vi "Main.vi"() -> ()   [LabVIEW 2016]
uses:
  SubVIS/MainSteps.ctl
  <vilib>/Utility/config.llb/Write Key (String).vi
  <vilib>/Utility/config.llb/Write Key (Double).vi
  <vilib>/Utility/config.llb/NI_LVConfig.lvlib
panel:
  out "全局图片":bool=TRUE
  out "新值":enum32{"三角形", "圆形", "正方形"}(ring)
  out "Status":bool
  in  "状态":string
  in  "标定":bool
  in  "停止":bool
  in  "运行":bool
  out "Image":T1(plugin-control)
  in  "选项卡控件":enum32{"三角形", "圆形", "正方形"}(tab)
  in  "Trangle保存":bool
  in  "Trangle打开":bool
  in  "Trangle参考":bool
  in  "多列列表框":i32(listbox)
  in  "Trangle处理":bool
  in  "Point1":cluster{"伺服X":dbl, "伺服Y":dbl}
  in  "Point2":cluster{"伺服X":dbl, "伺服Y":dbl}
  in  "Point3":cluster{"伺服X":dbl, "伺服Y":dbl}
  in  "Mark":cluster{"伺服X":dbl, "伺服Y":dbl}
  in  "半径R":dbl
  in  "Circle参考":bool
  in  "Circle打开":bool
  in  "多列列表框":i32(listbox) caption="圆形"
  in  "Circle保存":bool
  in  "Circle处理":bool
  in  "Mark":cluster{"伺服X":dbl, "伺服Y":dbl}
  in  "Mark":cluster{"伺服X":dbl, "伺服Y":dbl}
  in  "Point4":cluster{"伺服X":dbl, "伺服Y":dbl}
  in  "Point3":cluster{"伺服X":dbl, "伺服Y":dbl}
  in  "Point2":cluster{"伺服X":dbl, "伺服Y":dbl}
  in  "Point1":cluster{"伺服X":dbl, "伺服Y":dbl}
  in  "Square处理":bool
  in  "多列列表框":i32(listbox) caption="正方形"
  in  "Square参考":bool
  in  "Square打开":bool
  in  "Square保存":bool
  # "湖南工业大学毕设视觉平台"
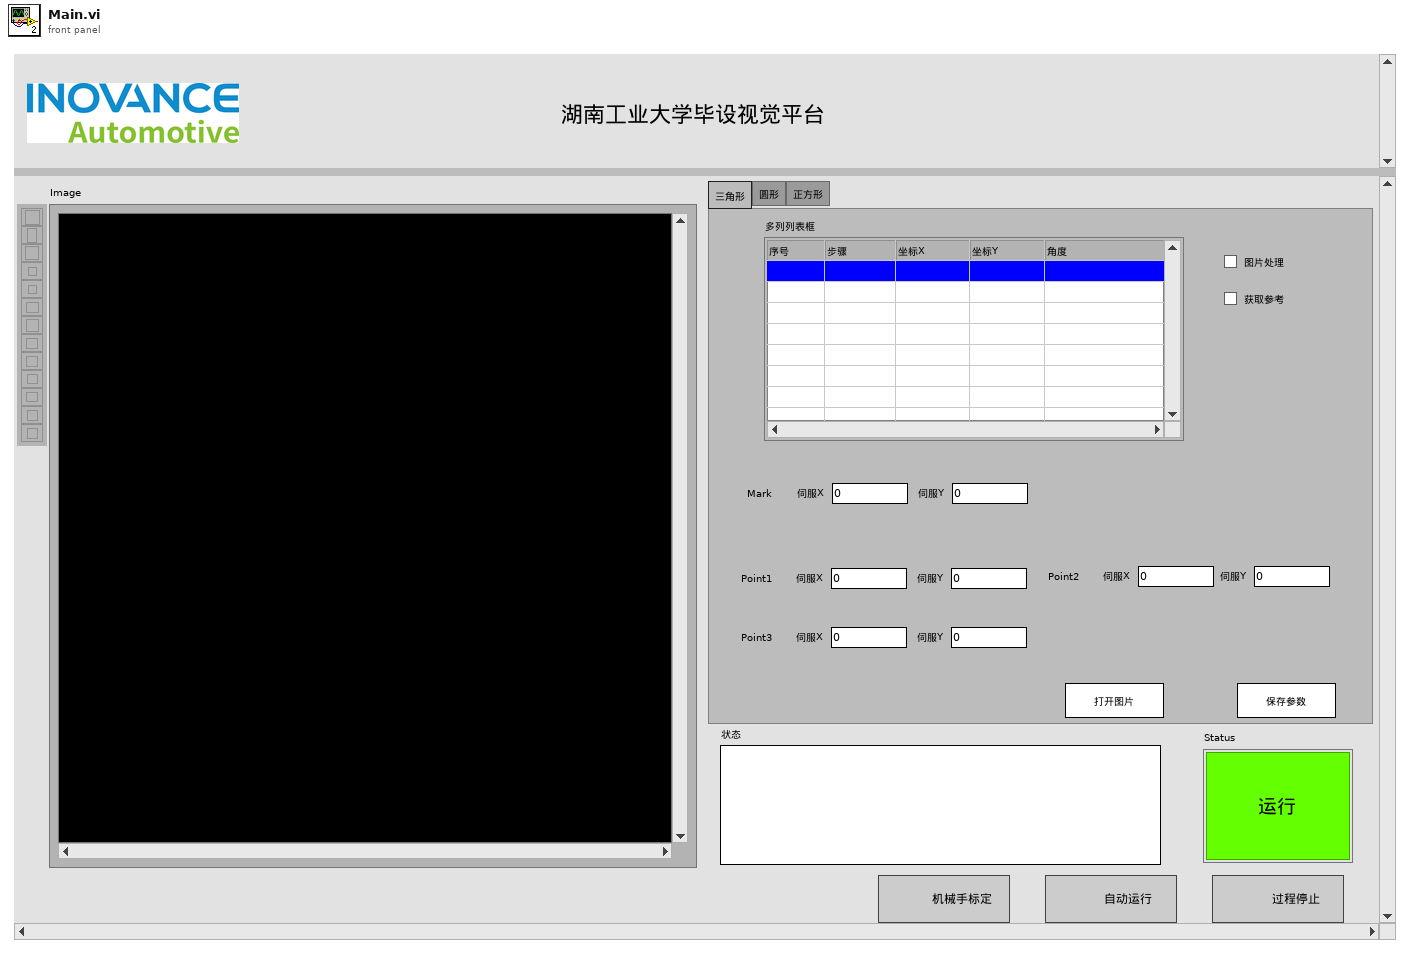
[diagram p1: front panel]
types:
  T1 = typedef "IMAQ Image.ctl" = refnum<image>
  T2 = typedef "MainSteps.ctl" = enum16{"Nothing", "Initial", "ReadConfig", "OpenPicture", "PicturePro", "SaveRefer", "SaveParam", "AutoRun", "Exit"}
  T3 = typedef "Image Type" = u32
  T4 = typedef "NI_LVConfig.lvlib/Config Data RefNum.ctl" = refnum<k1>
  T5 = cluster{"Center (Pixels)":cluster{"X":sgl, "Y":sgl}, "Radius (Pixels)":dbl, "Center (Real-World)":cluster{"X":sgl, "Y":sgl}, "Radius (Real-World)":dbl, "Roundness (Real-World)":dbl, "Average Strength":dbl, "Average SNR (dB)":dbl}
  T6 = cluster{"Position":cluster{"x":sgl, "y":sgl}, "Angle":sgl, "Scale":sgl, "Score":sgl, "Bounding Box":cluster{"x":sgl, "y":sgl}[]}[]
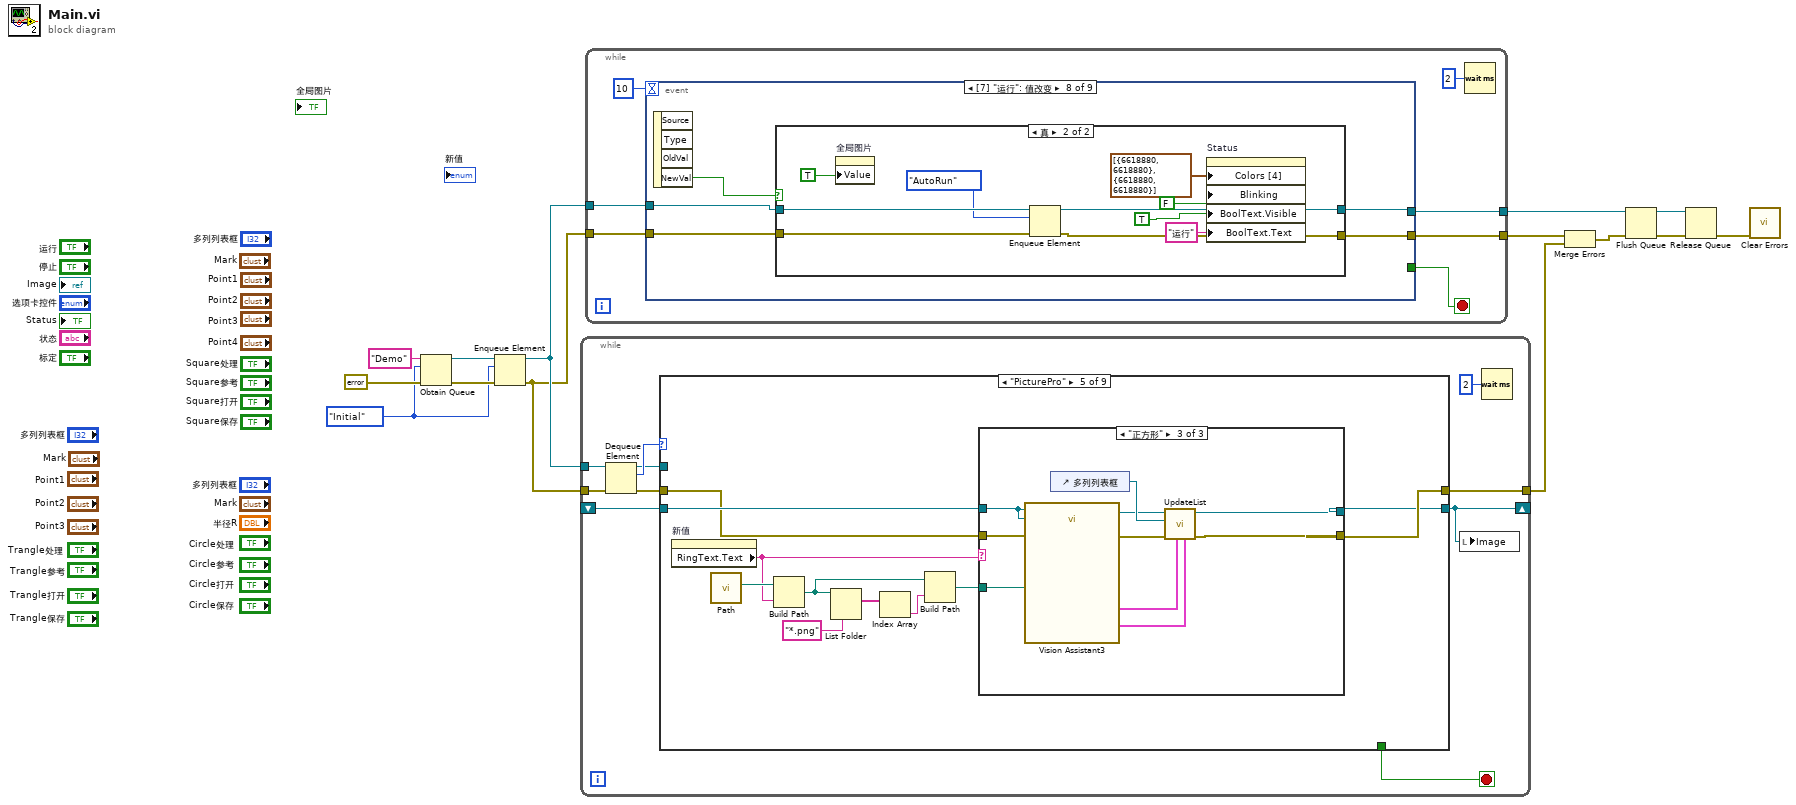
[diagram p0: block diagram]
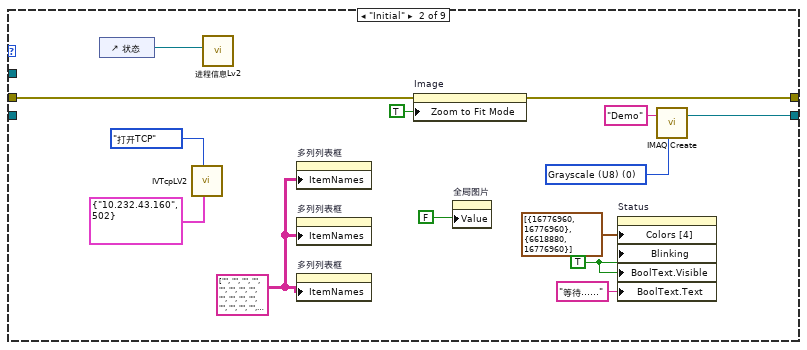
[diagram p3: hidden frame]
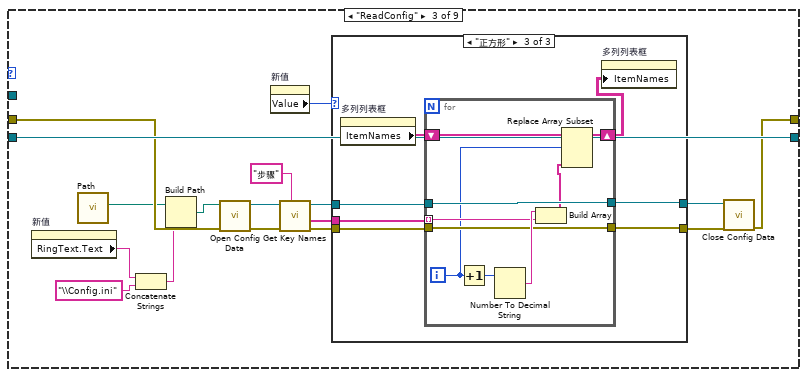
[diagram p4: hidden frame]
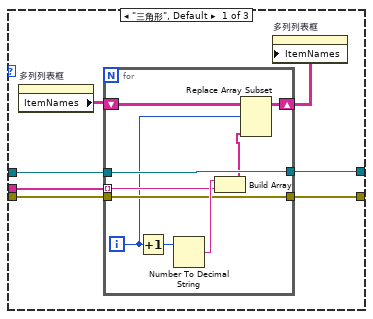
[diagram p5: hidden frame]
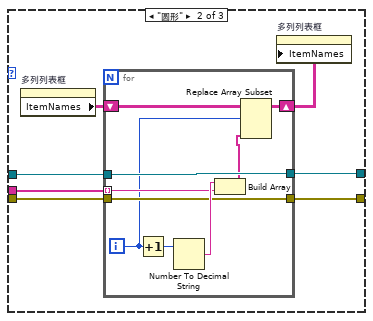
[diagram p6: hidden frame]
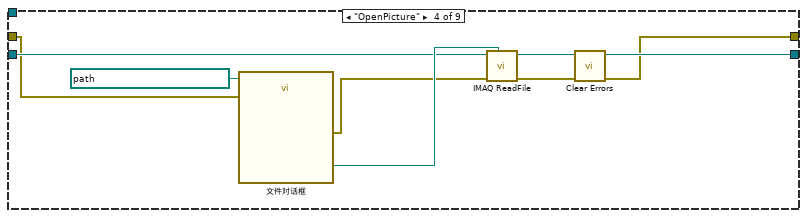
[diagram p7: hidden frame]
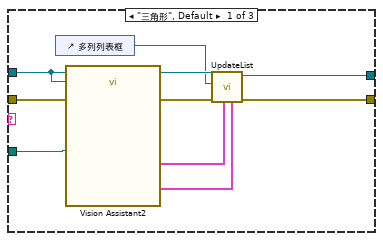
[diagram p8: hidden frame]
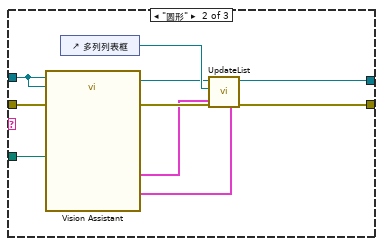
[diagram p9: hidden frame]
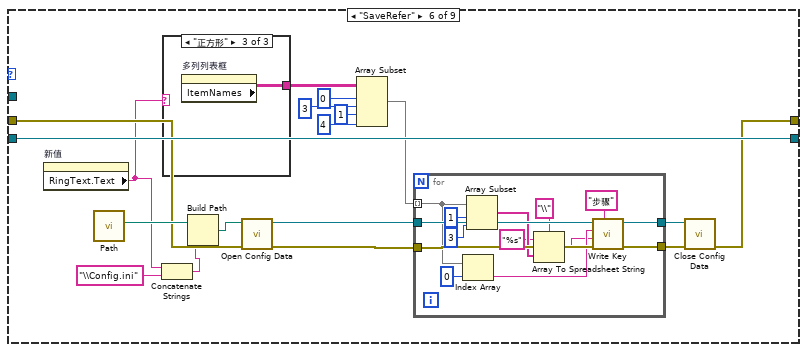
[diagram p10: hidden frame]
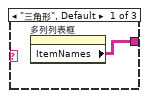
[diagram p11: hidden frame]
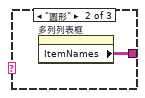
[diagram p12: hidden frame]
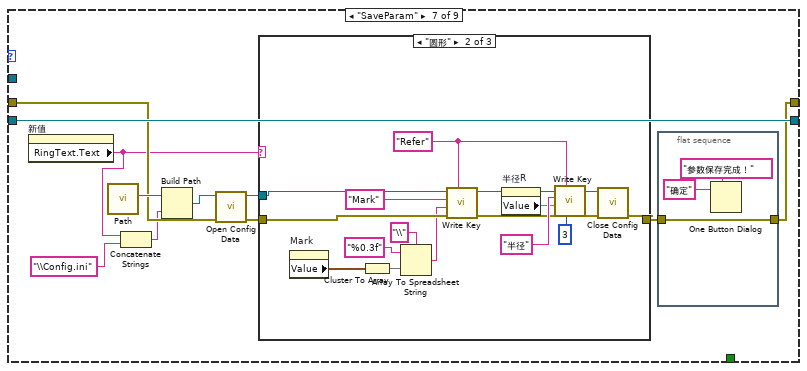
[diagram p13: hidden frame]
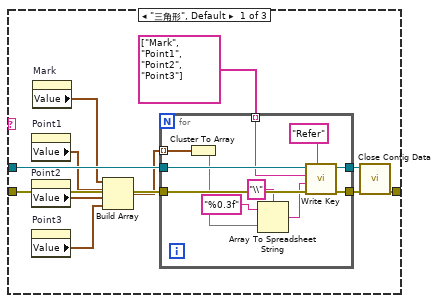
[diagram p14: hidden frame]
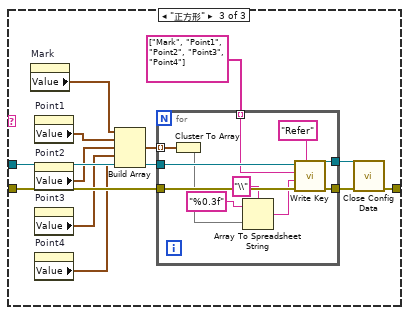
[diagram p15: hidden frame]
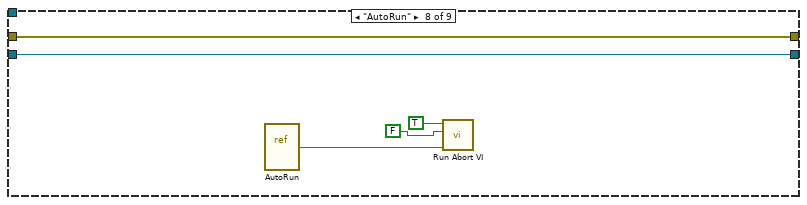
[diagram p16: hidden frame]
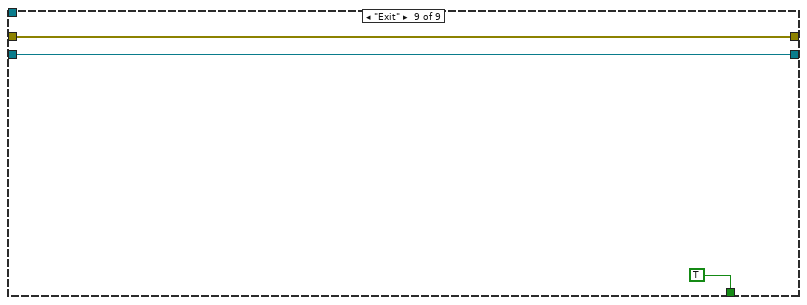
[diagram p17: hidden frame]
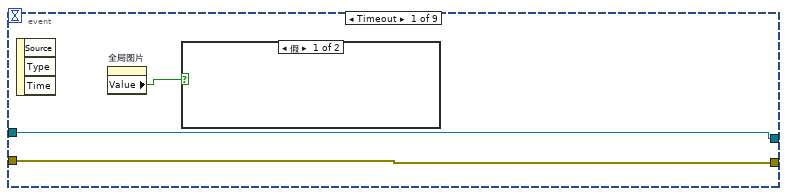
[diagram p18: hidden frame]
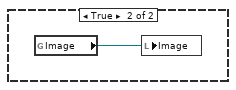
[diagram p19: hidden frame]
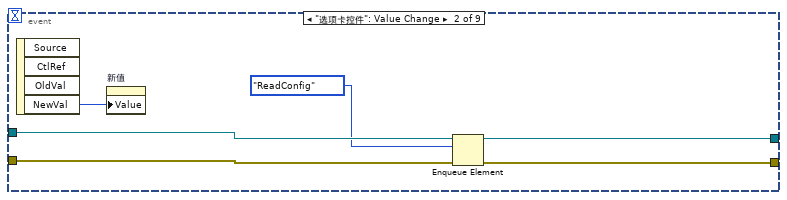
[diagram p20: hidden frame]
diagram:
  w9 = MainSteps."Initial"
  n1 = Obtain Queue(name (unnamed)="Demo" ("名称（未命名）"), element data type=w9, error in (no error)=errorcluster {"status"=FALSE, "code"=0, "source"=""} ("错误输入（无错误）")) -> (queue out=w13:refnum<queue>, error out=w12:errorcluster)  [unwired: 2 in, 1 out]
  n2 = Enqueue Element(queue=w13, element=w9, error in (no error)=w12) -> (queue out=w10:refnum<queue>, error out=w8:errorcluster)  [unwired: 1 in, 1 out]
  n3 = while {
    tunnel: w8 -> [w24]
    tunnel: w10 -> [w23]
    shift-right: [w16] -> _
    shift-left: _ -> [w19]
    tunnel: [w18] -> w6
    stop <- w17 stop-if-true
    n4 = Dequeue Element(queue=w23, error in (no error)=w24) -> (queue out=w21:refnum<queue>, element=w22:T2, error out=w20:errorcluster)  [unwired: 1 in, 1 out]
    n5 = case shown="\"PicturePro\"" w22 {
      tunnel: w21 -> [_ _ _ _ _ _ _ _ _]
      tunnel: w20 -> [w26 w37 w56 w109 w123 w169 w197 w270 w273]
      tunnel: [w25 w39 w57 w110 w121 w172 w200 w269 w272] -> w16
      tunnel: w19 -> [w25 _ w57 w111 w124 w172 w200 w269 w272]
      tunnel: [w26 w36 w45 w106 w122 w158 w193 w270 w273] -> w18
      tunnel: [_ _ _ _ _ _ _ _ TRUE] -> w17
      frame "Nothing", Default {
      }
      frame "Initial" {
        w28 = TRUE ("闪烁")
        w34 = T3 0 items=["Grayscale (U8)", "Grayscale (I16)", "Grayscale (SGL)", "Complex (CSG)", "RGB (U32)", "HSL (U32)", "RGB (U64)", "Grayscale (U16)"] ("Image Type")
        w38 = string[][] [["", "", "", "", "", ""], ["", "", "", "", "", ""], ["", "", "", "", "", ""], ["", "", "", "", "", ""], ["", "", "", "", "", ""], ["", "", "", "", "", " "]] ("项名")
        n6 = control-ref of="状态"() -> (w33:refnum<vi>)
        n7 = call "IVTcpLV2.vi"("TCP连接参数"=cluster{"IP地址":string, "端口":u16} {"IP地址"="10.232.43.160", "端口"=502}, "TCP操作模式"=enum16{"打开TCP", "读MW区", "写MW区", "关闭TCP"}."打开TCP") -> ()  [unwired: 6 in, 4 out]
        n8 = call "进程信息Lv2.vi"("进程状态"=w33) -> ()  [unwired: 6 in, 1 out]
        n9 = property on="多列列表框" class="MCListbox (严格)"("ItemNames"=w38) -> ()  [unwired: 2 in, 2 out]
        n10 = property on="多列列表框" class="MCListbox (严格)"("ItemNames"=w38) -> ()  [unwired: 2 in, 2 out]
        n11 = property on="多列列表框" class="MCListbox (严格)"("ItemNames"=w38) -> ()  [unwired: 2 in, 2 out]
        n12 = property on="Image" class="ImageControl"(error in=w37, "Zoom to Fit Mode"=TRUE) -> (error out=w36:errorcluster)  [unwired: 1 in, 1 out]
        n13 = property on="全局图片" class="Bool (严格)"("Value"=FALSE) -> ()  [unwired: 2 in, 2 out]
        n14 = property on="Status" class="Bool (严格)"("Colors [4]"=cluster{u32, u32}[] [{16776960, 16776960}, {6618880, 16776960}] ("颜色[4]"), "Blinking"=w28, "BoolText.Visible"=w28, "BoolText.Text"="等待……" ("布尔文本.文本")) -> ()  [unwired: 2 in, 2 out]
        n15 = call "IMAQ Create"("Image Name"="Demo", "Image Type"=w34) -> ("New Image"=w39:T1)  [unwired: 3 in, 1 out]
      }
      frame "ReadConfig" {
        n16 = property on="新值" class="Enum (严格)"() -> ("RingText.Text"=w41:string)  [unwired: 2 in, 2 out]
        n17 = call "Path.vi"() -> ("Total"=w52:path)  [unwired: 11 in]
        n18 = Concatenate Strings(w41, "\\Config.ini" ("section")) -> (w42:string)
        n19 = Build Path(base path=w52, name or relative path=w42) -> (appended path=w51:path)
        n20 = call <vilib>:"Open Config Data.vi"("error in (no error)"=w56, "configuration file path"=w51) -> ("error out"=w54:errorcluster, "refnum"=w55:T4)  [unwired: 7 in, 1 out]
        n21 = property on="新值" class="Enum (严格)"() -> ("Value"=w44:enum32{"三角形", "圆形", "正方形"})  [unwired: 2 in, 2 out]
        n22 = call <vilib>:"Get Key Names.vi"("section"="步骤", "error in (no error)"=w54, "refnum"=w55) -> ("error out"=w50:errorcluster, "key names"=w49:string[], "refnum out"=w48:T4)  [unwired: 5 in, 1 out]
        n23 = case shown="\"正方形\"" w44 {
          tunnel: w50 -> [w64 w80 w96]
          tunnel: w49 -> [w63 w79 w93]
          tunnel: w48 -> [w60 w78 w94]
          tunnel: [w61 w77 w92] -> w47
          tunnel: [w62 w76 w95] -> w46
          frame "三角形", Default {
            n24 = property on="多列列表框" class="MCListbox (严格)"() -> ("ItemNames"=w59:string[][])  [unwired: 2 in, 2 out]
            n25 = for {
              tunnel: w64 -> [w69]
              tunnel: w63 -> [w71] mode=indexing
              tunnel: w60 -> [w70]
              tunnel: [w70] -> w61
              tunnel: [w69] -> w62
              shift-right: [w65] -> w58
              shift-left: w59 -> [w68]
              i -> [w67]
              n26 = Increment(x=w67) -> (x+1=w73:i32)
              n27 = Number To Decimal String(number=w73) -> (decimal integer string=w72:string)  [unwired: 1 in]
              n28 = Build Array(w72, w71) -> (w66:string[])
              n29 = Replace Array Subset(array=w68, new element=w66, index (row)=w67) -> (w65:string[][])  [unwired: 1 in]
            }
            n30 = property on="多列列表框" class="MCListbox (严格)"("ItemNames"=w58) -> ()  [unwired: 2 in, 2 out]
          }
          frame "圆形" {
            n31 = property on="多列列表框" class="MCListbox (严格)"() -> ("ItemNames"=w75:string[][])  [unwired: 2 in, 2 out]
            n32 = for {
              tunnel: w80 -> [w85]
              tunnel: w79 -> [w87] mode=indexing
              tunnel: w78 -> [w86]
              tunnel: [w86] -> w77
              tunnel: [w85] -> w76
              shift-right: [w81] -> w74
              shift-left: w75 -> [w84]
              i -> [w83]
              n33 = Increment(x=w83) -> (x+1=w89:i32)
              n34 = Number To Decimal String(number=w89) -> (decimal integer string=w88:string)  [unwired: 1 in]
              n35 = Build Array(w88, w87) -> (w82:string[])
              n36 = Replace Array Subset(array=w84, new element=w82, index (row)=w83) -> (w81:string[][])  [unwired: 1 in]
            }
            n37 = property on="多列列表框" class="MCListbox (严格)"("ItemNames"=w74) -> ()  [unwired: 2 in, 2 out]
          }
          frame "正方形" {
            n38 = property on="多列列表框" class="MCListbox (严格)"() -> ("ItemNames"=w91:string[][])  [unwired: 2 in, 2 out]
            n39 = for {
              tunnel: w96 -> [w101]
              tunnel: w93 -> [w103] mode=indexing
              tunnel: w94 -> [w102]
              tunnel: [w102] -> w92
              tunnel: [w101] -> w95
              shift-right: [w97] -> w90
              shift-left: w91 -> [w100]
              i -> [w99]
              n40 = Increment(x=w99) -> (x+1=w105:i32)
              n41 = Number To Decimal String(number=w105) -> (decimal integer string=w104:string)  [unwired: 1 in]
              n42 = Build Array(w104, w103) -> (w98:string[])
              n43 = Replace Array Subset(array=w100, new element=w98, index (row)=w99) -> (w97:string[][])  [unwired: 1 in]
            }
            n44 = property on="多列列表框" class="MCListbox (严格)"("ItemNames"=w90) -> ()  [unwired: 2 in, 2 out]
          }
        }
        n45 = call <vilib>:"Close Config Data.vi"("error in (no error)"=w46, "refnum"=w47) -> ("error out"=w45:errorcluster)  [unwired: 8 in, 1 out]
      }
      frame "OpenPicture" {
        n46 = call "文件对话框"("start path"=path "E:/项目/湖南工业大学/图片", "error in"=w109) -> ("selected path"=w112:path, "error out"=w108:errorcluster)  [unwired: 10 in, 2 out]
        n47 = call "IMAQ ReadFile"("File Path"=w112, "error in (no error)"=w108, "Image"=w111) -> ("error out"=w107:errorcluster, "Image Out"=w110:T1)  [unwired: 4 in, 3 out]
        n48 = call <vilib>:"Clear Errors.vi"("error in (no error)"=w107) -> ("error out"=w106:errorcluster)  [unwired: 5 in, 1 out]
      }
      frame "PicturePro" {
        n49 = property on="新值" class="Enum (严格)"() -> ("RingText.Text"=w115:string)  [unwired: 2 in, 2 out]
        n50 = call "Path.vi"() -> ("Total"=w116:path)  [unwired: 11 in]
        n51 = Build Path(base path=w116, name or relative path=w115) -> (appended path=w114:path)
        n52 = List Folder(path=w114, pattern="*.png" ("类型")) -> (filenames=w120:string[])  [unwired: 2 in, 3 out]
        n53 = Index Array(array=w120) -> (element=w119:string)  [unwired: 1 in]
        n54 = Build Path(base path=w114, name or relative path=w119) -> (appended path=w118:path)
        n55 = case shown="\"正方形\"" w115 {
          tunnel: w124 -> [w133 w144 w154]
          tunnel: w123 -> [w132 w143 w153]
          tunnel: [w130 w142 w150] -> w122
          tunnel: [w127 w141 w146] -> w121
          tunnel: w118 -> [w134 w140 w152]
          frame "三角形", Default {
            n56 = control-ref of="多列列表框"() -> (w126:refnum<vi>)
            n57 = call "Vision Assistant2"("Image In"=w133, "Image Dst"=w133, "Template File Path (Pattern Matching 1)"=w134, "error in"=w132) -> ("Image Out"=w128:T1, "Fitted Circle (Find Circular Edge 1)"=w125:T5, "Matches (Pattern Matching 1)"=w129:T6, "error out"=w131:errorcluster)  [unwired: 20 in]
            n58 = call "UpdateList.vi"("Fitted Circle (Find Circular Edge 1)"=w125, "Matches"=w129, "错误输入"=w131, "MCListbox引用句柄"=w126, "Image in"=w128) -> ("错误输出"=w130:errorcluster, "Image out"=w127:T1)  [unwired: 5 in]
          }
          frame "圆形" {
            n59 = call "Vision Assistant"("Image In"=w144, "Image Dst"=w144, "Template File Path (Pattern Matching 1)"=w140, "error in"=w143) -> ("Image Out"=w136:T1, "Fitted Circle (Find Circular Edge 1)"=w135:T5, "Matches (Pattern Matching 1)"=w138:T6, "error out"=w139:errorcluster)  [unwired: 20 in]
            n60 = control-ref of="多列列表框"() -> (w137:refnum<vi>)
            n61 = call "UpdateList.vi"("Fitted Circle (Find Circular Edge 1)"=w135, "Matches"=w138, "错误输入"=w139, "MCListbox引用句柄"=w137, "Image in"=w136) -> ("错误输出"=w142:errorcluster, "Image out"=w141:T1)  [unwired: 5 in]
          }
          frame "正方形" {
            n62 = call "Vision Assistant3"("Image In"=w154, "Image Dst"=w154, "Template File Path (Pattern Matching 1)"=w152, "error in"=w153) -> ("Image Out"=w147:T1, "Fitted Circle (Find Circular Edge 1)"=w145:T5, "Matches (Pattern Matching 1)"=w149:T6, "error out"=w151:errorcluster)  [unwired: 20 in]
            n63 = control-ref of="多列列表框"() -> (w148:refnum<vi>)
            n64 = call "UpdateList.vi"("Fitted Circle (Find Circular Edge 1)"=w145, "Matches"=w149, "错误输入"=w151, "MCListbox引用句柄"=w148, "Image in"=w147) -> ("错误输出"=w150:errorcluster, "Image out"=w146:T1)  [unwired: 5 in]
          }
        }
      }
      frame "SaveRefer" {
        n65 = property on="新值" class="Enum (严格)"() -> ("RingText.Text"=w156:string)  [unwired: 2 in, 2 out]
        n66 = call "Path.vi"() -> ("Total"=w171:path)  [unwired: 11 in]
        n67 = Concatenate Strings(w156, "\\Config.ini" ("section")) -> (w155:string)
        n68 = case shown="\"正方形\"" w156 {
          tunnel: [w173 w174 w175] -> w163
          frame "三角形", Default {
            n69 = property on="多列列表框" class="MCListbox (严格)"() -> ("ItemNames"=w173:string[][])  [unwired: 2 in, 2 out]
          }
          frame "圆形" {
            n70 = property on="多列列表框" class="MCListbox (严格)"() -> ("ItemNames"=w174:string[][])  [unwired: 2 in, 2 out]
          }
          frame "正方形" {
            n71 = property on="多列列表框" class="MCListbox (严格)"() -> ("ItemNames"=w175:string[][])  [unwired: 2 in, 2 out]
          }
        }
        n72 = Build Path(base path=w171, name or relative path=w155) -> (appended path=w170:path)
        n73 = call <vilib>:"Open Config Data.vi"("error in (no error)"=w169, "configuration file path"=w170) -> ("error out"=w167:errorcluster, "refnum"=w168:T4)  [unwired: 7 in, 1 out]
        n74 = Array Subset(array=w163, index (row)=0 ("索引"), length (row)=3 ("索引"), index (col)=1 ("索引"), length (col)=4 ("索引")) -> (w166:string[][])
        n75 = for {
          tunnel: w168 -> [w188]
          tunnel: w167 -> [w187]
          tunnel: w166 -> [w184] mode=indexing
          tunnel: [w177] -> w165
          tunnel: [w176] -> w164
          n76 = Index Array(array=w184, index=0 ("索引")) -> (element=w185:string)
          n77 = Array Subset(array=w184, index=1 ("索引"), length=3 ("长度")) -> (w181:string[])
          n78 = Array To Spreadsheet String(delimiter (Tab)="\\" ("分隔符(Tab)"), array=w181, 3:"%s" ("格式字符串")) -> (spreadsheet string=w178:string)
          n79 = call-poly <vilib>:"Write Key.vi"("section"="步骤", "error in (no error)"=w187, "value"=w178, "key"=w185, "refnum"=w188) -> ("error out"=w176:errorcluster, "refnum out"=w177:T4)  [unwired: 4 in, 1 out]
        }
        n80 = call <vilib>:"Close Config Data.vi"("error in (no error)"=w164, "refnum"=w165) -> ("error out"=w158:errorcluster)  [unwired: 8 in, 1 out]
      }
      frame "SaveParam" {
        n81 = property on="新值" class="Enum (严格)"() -> ("RingText.Text"=w190:string)  [unwired: 2 in, 2 out]
        n82 = call "Path.vi"() -> ("Total"=w199:path)  [unwired: 11 in]
        n83 = Concatenate Strings(w190, "\\Config.ini" ("section")) -> (w192:string)
        n84 = Build Path(base path=w199, name or relative path=w192) -> (appended path=w198:path)
        n85 = call <vilib>:"Open Config Data.vi"("error in (no error)"=w197, "configuration file path"=w198) -> ("error out"=w195:errorcluster, "refnum"=w196:T4)  [unwired: 7 in, 1 out]
        n86 = case shown="\"圆形\"" w190 {
          tunnel: w196 -> [w213 w231 w253]
          tunnel: w195 -> [w212 w234 w254]
          tunnel: [w206 w239 w244] -> w194
          frame "三角形", Default {
            n87 = property on="Point1" class="Clust (严格)"() -> ("Value"=w211:cluster{"伺服X":dbl, "伺服Y":dbl})  [unwired: 2 in, 2 out]
            n88 = property on="Point2" class="Clust (严格)"() -> ("Value"=w209:cluster{"伺服X":dbl, "伺服Y":dbl})  [unwired: 2 in, 2 out]
            n89 = property on="Point3" class="Clust (严格)"() -> ("Value"=w210:cluster{"伺服X":dbl, "伺服Y":dbl})  [unwired: 2 in, 2 out]
            n90 = property on="Mark" class="Clust (严格)"() -> ("Value"=w204:cluster{"伺服X":dbl, "伺服Y":dbl})  [unwired: 2 in, 2 out]
            n91 = Build Array(w204, w211, w209, w210) -> (w208:cluster{"伺服X":dbl, "伺服Y":dbl}[])
            n92 = for {
              tunnel: w212 -> [w225]
              tunnel: w213 -> [w224]
              tunnel: w208 -> [w222] mode=indexing
              tunnel: [w221] -> w207
              tunnel: string[] ["Mark", "Point1", "Point2", "Point3"] -> [w220] mode=indexing
              tunnel: [w215] -> w205
              n93 = Cluster To Array(cluster=w222) -> (array=w219:dbl[])
              n94 = Array To Spreadsheet String(delimiter (Tab)="\\" ("分隔符(Tab)"), array=w219, 3:"%0.3f" ("分隔符(Tab)")) -> (spreadsheet string=w216:string)
              n95 = call-poly <vilib>:"Write Key.vi"("section"="Refer", "error in (no error)"=w225, "value"=w216, "key"=w220, "refnum"=w224) -> ("error out"=w221:errorcluster, "refnum out"=w215:T4)  [unwired: 4 in, 1 out]
            }
            n96 = call <vilib>:"Close Config Data.vi"("error in (no error)"=w207, "refnum"=w205) -> ("error out"=w206:errorcluster)  [unwired: 8 in, 1 out]
          }
          frame "圆形" {
            w229 = "Refer" ("section")
            n97 = property on="Mark" class="Clust (严格)"() -> ("Value"=w226:cluster{"伺服X":dbl, "伺服Y":dbl})  [unwired: 2 in, 2 out]
            n98 = Cluster To Array(cluster=w226) -> (array=w227:dbl[])
            n99 = Array To Spreadsheet String(delimiter (Tab)="\\" ("分隔符(Tab)"), array=w227, 3:"%0.3f" ("分隔符(Tab)")) -> (spreadsheet string=w230:string)
            n100 = call-poly <vilib>:"Write Key.vi"("section"=w229, "error in (no error)"=w234, "value"=w230, "key"="Mark" ("section"), "refnum"=w231) -> ("error out"=w233:errorcluster, "refnum out"=w232:T4)  [unwired: 4 in, 1 out]
            n101 = property on="半径R" class="DigNum (严格)"() -> ("Value"=w241:dbl)  [unwired: 2 in, 2 out]
            n102 = call-poly <vilib>:"Write Key.vi"("precision (6)"=i16 3, "section"=w229, "error in (no error)"=w233, "value"=w241, "key"="半径", "refnum"=w232) -> ("error out"=w240:errorcluster, "refnum out"=w238:T4)  [unwired: 3 in, 1 out]
            n103 = call <vilib>:"Close Config Data.vi"("error in (no error)"=w240, "refnum"=w238) -> ("error out"=w239:errorcluster)  [unwired: 8 in, 1 out]
          }
          frame "正方形" {
            n104 = property on="Mark" class="Clust (严格)"() -> ("Value"=w243:cluster{"伺服X":dbl, "伺服Y":dbl})  [unwired: 2 in, 2 out]
            n105 = property on="Point1" class="Clust (严格)"() -> ("Value"=w252:cluster{"伺服X":dbl, "伺服Y":dbl})  [unwired: 2 in, 2 out]
            n106 = property on="Point2" class="Clust (严格)"() -> ("Value"=w251:cluster{"伺服X":dbl, "伺服Y":dbl})  [unwired: 2 in, 2 out]
            n107 = property on="Point3" class="Clust (严格)"() -> ("Value"=w250:cluster{"伺服X":dbl, "伺服Y":dbl})  [unwired: 2 in, 2 out]
            n108 = property on="Point4" class="Clust (严格)"() -> ("Value"=w249:cluster{"伺服X":dbl, "伺服Y":dbl})  [unwired: 2 in, 2 out]
            n109 = Build Array(w243, w252, w251, w250, w249) -> (w248:cluster{"伺服X":dbl, "伺服Y":dbl}[])
            n110 = for {
              tunnel: w254 -> [w265]
              tunnel: w253 -> [w264]
              tunnel: w248 -> [w262] mode=indexing
              tunnel: [w261] -> w245
              tunnel: string[] ["Mark", "Point1", "Point2", "Point3", "Point4"] -> [w260] mode=indexing
              tunnel: [w255] -> w246
              n111 = Cluster To Array(cluster=w262) -> (array=w259:dbl[])
              n112 = Array To Spreadsheet String(delimiter (Tab)="\\" ("分隔符(Tab)"), array=w259, 3:"%0.3f" ("分隔符(Tab)")) -> (spreadsheet string=w256:string)
              n113 = call-poly <vilib>:"Write Key.vi"("section"="Refer", "error in (no error)"=w265, "value"=w256, "key"=w260, "refnum"=w264) -> ("error out"=w261:errorcluster, "refnum out"=w255:T4)  [unwired: 4 in, 1 out]
            }
            n114 = call <vilib>:"Close Config Data.vi"("error in (no error)"=w245, "refnum"=w246) -> ("error out"=w244:errorcluster)  [unwired: 8 in, 1 out]
          }
        }
        n115 = flat-sequence {
          tunnel: w194 -> [w203]
          tunnel: [w203] -> w193
          frame #0 {
            n116 = One Button Dialog(message="参数保存完成！" ("消息"), button name ("OK")="确定" ("按钮名称（“确定”）")) -> ()  [unwired: 1 out]
          }
        }
      }
      frame "AutoRun" {
        n117 = vi-ref "AutoRun.vi"() -> (w268:refnum<vi>)
        n118 = call "Run Abort VI.vi"("VI引用句柄"=w268, "Front Panel Window:Open"=FALSE ("Run?(Default Abort)"), "Run?(Default Abort)"=TRUE) -> ()  [unwired: 9 in]
      }
      frame "Exit" {
      }
    }
    n119 = local write "Image"(w16) -> ()
    n120 = Wait (ms)(milliseconds to wait=u32 2 ("等待时间（毫秒）")) -> ()  [unwired: 1 out]
  }
  n121 = while {
    tunnel: w10 -> [w279]
    tunnel: w8 -> [w278]
    tunnel: [w277] -> w3
    tunnel: [w276] -> w7
    stop <- w275 stop-if-true
    n122 = event shown="[7] \"运行\": 值改变" {
      selector: _ -> [_ _ _ _ _ _ _ _ _]
      dyn-events: _ -> [_ _ _ _ _ _ _ _ _]
      timeout: 10 -> [_ _ _ _ _ _ _ _ _]
      tunnel: w279 -> [w283 w290 w293 w304 w318 w330 w343 w345 w365]
      tunnel: w278 -> [w282 w288 w295 w303 w315 w329 w342 w347 w364]
      tunnel: [w283 w289 w291 w306 w317 w328 w343 w344 w363] -> w277
      tunnel: [w282 w287 w294 w305 w316 w327 w342 w346 w362] -> w276
      tunnel: [_ _ _ _ _ _ _ _ w361] -> w275
      event Timeout {
        n123 = event-data() -> ()  [unwired: 1 in, 3 out]
        n124 = property on="全局图片" class="Bool (严格)"() -> ("Value"=w281:bool)  [unwired: 2 in, 2 out]
        n125 = case shown="假" w281 {
          frame False {
          }
          frame True {
            n126 = global read "全局.vi" "Image"() -> (w284:T1)
            n127 = local write "Image"(w284) -> ()
          }
        }
      }
      event "选项卡控件": Value Change {
        n128 = event-data() -> ("NewVal"=w285:enum32{"三角形", "圆形", "正方形"})  [unwired: 1 in, 3 out]
        n129 = property on="新值" class="Enum (严格)"("Value"=w285) -> ()  [unwired: 2 in, 2 out]
        n130 = Enqueue Element(queue=w290, element=MainSteps."ReadConfig", error in (no error)=w288) -> (queue out=w289:refnum<queue>, error out=w287:errorcluster)  [unwired: 1 in, 1 out]
      }
      event "Trangle打开", "Square打开", "Circle打开": Value Change {
        n131 = event-data() -> ("NewVal"=w292:bool)  [unwired: 1 in, 3 out]
        n132 = case shown="真" w292 {
          tunnel: w295 -> [w296 w302]
          tunnel: [w296 w301] -> w294
          tunnel: w293 -> [w297 w300]
          tunnel: [w297 w298] -> w291
          frame False {
          }
          frame True {
            n133 = Enqueue Element(queue=w300, element=MainSteps."OpenPicture", error in (no error)=w302) -> (queue out=w298:refnum<queue>, error out=w301:errorcluster)  [unwired: 1 in, 1 out]
          }
        }
      }
      event "Square处理", "Circle处理", "Trangle处理": Value Change {
        n134 = event-data() -> ("NewVal"=w307:bool)  [unwired: 1 in, 3 out]
        n135 = case shown="真" w307 {
          tunnel: [w309 w314] -> w306
          tunnel: [w308 w313] -> w305
          tunnel: w304 -> [w309 w312]
          tunnel: w303 -> [w308 w311]
          frame False {
          }
          frame True {
            n136 = Enqueue Element(queue=w312, element=MainSteps."PicturePro", error in (no error)=w311) -> (queue out=w314:refnum<queue>, error out=w313:errorcluster)  [unwired: 1 in, 1 out]
          }
        }
      }
      event "Square参考", "Circle参考", "Trangle参考": Value Change {
        n137 = event-data() -> ("NewVal"=w319:bool)  [unwired: 1 in, 3 out]
        n138 = case shown="真" w319 {
          tunnel: w318 -> [w321 w326]
          tunnel: [w321 w325] -> w317
          tunnel: [w320 w324] -> w316
          tunnel: w315 -> [w320 w323]
          frame False {
          }
          frame True {
            n139 = Enqueue Element(queue=w326, element=MainSteps."SaveRefer", error in (no error)=w323) -> (queue out=w325:refnum<queue>, error out=w324:errorcluster)  [unwired: 1 in, 1 out]
          }
        }
      }
      event "Circle保存", "Trangle保存", "Square保存": Value Change {
        n140 = event-data() -> ("NewVal"=w331:bool)  [unwired: 1 in, 3 out]
        n141 = case shown="假" w331 {
          tunnel: w330 -> [w333 w338]
          tunnel: w329 -> [w332 w337]
          tunnel: [w333 w336] -> w328
          tunnel: [w332 w335] -> w327
          frame False {
          }
          frame True {
            n142 = Enqueue Element(queue=w338, element=MainSteps."SaveParam", error in (no error)=w337) -> (queue out=w336:refnum<queue>, error out=w335:errorcluster)  [unwired: 1 in, 1 out]
          }
        }
      }
      event "标定": Value Change {
        n143 = event-data() -> ()  [unwired: 1 in, 4 out]
        n144 = vi-ref "相机标定-汇川机械手.vi"() -> (w341:refnum<vi>)
        n145 = call "Run Abort VI.vi"("VI引用句柄"=w341, "Front Panel Window:Open"=FALSE ("Run?(Default Abort)"), "Run?(Default Abort)"=TRUE) -> ()  [unwired: 9 in]
      }
      event "运行": Value Change {
        n146 = event-data() -> ("NewVal"=w348:bool)  [unwired: 1 in, 3 out]
        n147 = case shown="真" w348 {
          tunnel: w347 -> [w349 w360]
          tunnel: [w349 w359] -> w346
          tunnel: w345 -> [w350 w358]
          tunnel: [w350 w357] -> w344
          frame False {
          }
          frame True {
            n148 = property on="全局图片" class="Bool (严格)"("Value"=TRUE) -> ()  [unwired: 2 in, 2 out]
            n149 = Enqueue Element(queue=w358, element=MainSteps."AutoRun", error in (no error)=w360) -> (queue out=w357:refnum<queue>, error out=w359:errorcluster)  [unwired: 1 in, 1 out]
            n150 = property on="Status" class="Bool (严格)"("Colors [4]"=cluster{u32, u32}[] [{6618880, 6618880}, {6618880, 6618880}] ("颜色[4]"), "Blinking"=FALSE ("闪烁"), "BoolText.Visible"=TRUE ("闪烁"), "BoolText.Text"="运行" ("布尔文本.文本")) -> ()  [unwired: 2 in, 2 out]
          }
        }
      }
      event "停止": Value Change {
        n151 = event-data() -> ("NewVal"=w366:bool)  [unwired: 1 in, 3 out]
        n152 = case shown="真" w366 {
          tunnel: w365 -> [w368 w374]
          tunnel: w364 -> [w367 w373]
          tunnel: [w368 w371] -> w363
          tunnel: [w367 w370] -> w362
          tunnel: [_ TRUE] -> w361
          frame False {
          }
          frame True {
            n153 = Enqueue Element(queue=w374, element=MainSteps."Exit", error in (no error)=w373) -> (queue out=w371:refnum<queue>, error out=w370:errorcluster)  [unwired: 1 in, 1 out]
          }
        }
      }
    }
    n154 = Wait (ms)(milliseconds to wait=u32 2 ("等待时间（毫秒）")) -> ()  [unwired: 1 out]
  }
  n155 = Merge Errors(w7, w6) -> (w5:errorcluster)
  n156 = Flush Queue(queue=w3, error in (no error)=w5) -> (queue out=w2:refnum<queue>, error out=w4:errorcluster)  [unwired: 1 out]
  n157 = Release Queue(queue=w2, error in (no error)=w4) -> (error out=w1:errorcluster)  [unwired: 1 in, 2 out]
  n158 = call <vilib>:"Clear Errors.vi"("error in (no error)"=w1) -> ()  [unwired: 5 in, 2 out]
